vi "AI RT FIFO.vi"(0 "Data IN":dbl[](array[numeric]), 1 "Mode":T1=enum."Delete", 2 "AI RT FIFO Ref":refnum<vi>, 7 "Buffer Size":i32=10, 9 "# of elements":i32=1, 11 "Error IN":errorcluster, 12 "System Index":i32) -> (4 "Data OUT":dbl[][](array[numeric]), 6 "Empty?":bool, 8 "Size":i32, 15 "Error OUT":errorcluster)   [LabVIEW 2019]
uses:
  Type Defs and Controls/RT FIFO Mode.ctl
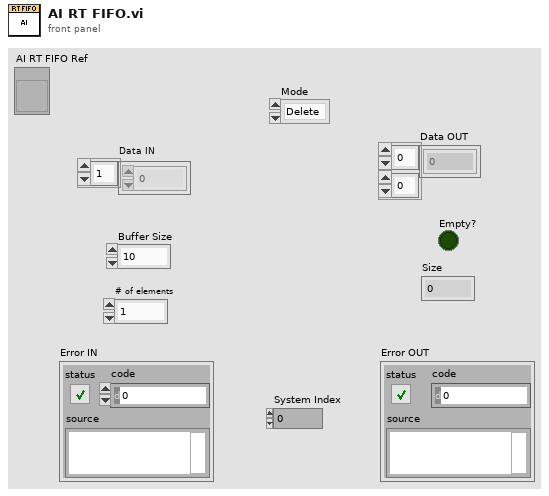
[diagram p1: front panel]
types:
  T1 = typedef "RT FIFO Mode.ctl" = enum16{"Create", "Write", "Read", "Delete"}
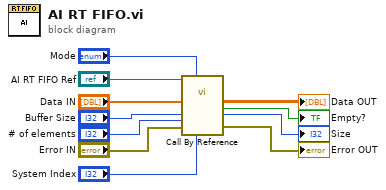
[diagram p0: block diagram]
diagram:
  n1 = call-by-ref "?"(reference="AI RT FIFO Ref", "Data IN"="Data IN", "Mode"="Mode", "Buffer Size"="Buffer Size", "# of elements"="# of elements", "Error IN"="Error IN", "System Index"="System Index") -> ("Data OUT"=→"Data OUT":dbl[][], "Empty?"=→"Empty?":bool, "Size"=→"Size":i32, "Error OUT"=→"Error OUT":errorcluster)  [unwired: 7 in, 2 out]
